vi "Add Element.vi"(8 "error in (no error)":errorcluster, 9 "Index (End)":i32=-1, 10 "Value":variant, 11 "ControlArray in":refnum<class "ControlArray.lvclass">) -> (0 "error out":errorcluster, 3 "ControlArray out":refnum<class "ControlArray.lvclass">)   [LabVIEW 2020, in "Control Array.lvlib" / "ControlArray.lvclass"]
uses:
  ControlArray.lvclass
  ControlArray.lvclass/ControlArray.ctl
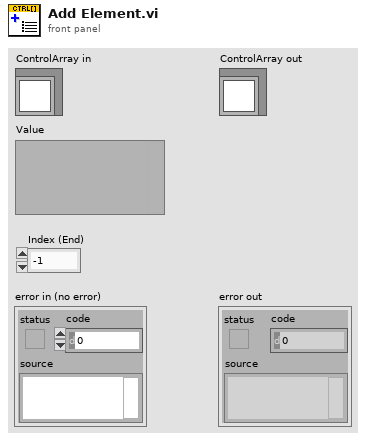
[diagram p1: front panel]
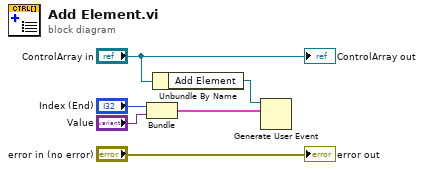
[diagram p0: block diagram]
diagram:
  n1 = Bundle("Index (End)"="Index (End)", "Value"="Value") -> (w1:cluster{"Index (End)":i32, "Value":variant})  [unwired: 1 in]
  n2 = Unbundle By Name("ControlArray in") -> ("Add Element"=w2:refnum<user-event>)
  n3 = Generate User Event(user event=w2, event data cluster=w1) -> ()  [unwired: 2 in, 2 out]
  "error out" <- "error in (no error)"
  "ControlArray out" <- "ControlArray in"
